vi "Handle Incoming Packets.vi"(8 "error in (no error)":errorcluster, 9 "SessionMailbox":refnum<queue>, 10 "Incoming Packet":refnum<class "ControlPacket.lvclass">, 11 "Server in":refnum<class "Server.lvclass">) -> (0 "error out":errorcluster, 1 "SessionMailbox out":refnum<queue>, 2 "Outgoing":T1, 3 "Server out":refnum<class "Server.lvclass">)   [LabVIEW 2013, in "MQTT Server.lvlib" / "Server.lvclass"]
uses:
  Server.lvclass
  Control Packets/ControlPacket/ControlPacket.lvclass
  MQTT_Base/Response -- cluster.ctl
  MQTT_Base/MQTT_Base.lvclass
  Control Packets/CONNECT/CONNECT.lvclass
  Control Packets/CONNACK/Connect Return Code -- enum.ctl
  Control Packets/PUBLISH/PUBLISH.lvclass
  Control Packets/ControlPacket/ControlPacket.lvclass/ControlPacket.ctl
  Control Packets/PUBREL/PUBREL.lvclass
  Control Packets/SUBSCRIBE/SUBSCRIBE.lvclass
  Control Packets/SUBACK/Subscription Success Code.ctl
  Control Packets/ControlPacket/QualityOfService -- enum.ctl
  Control Packets/UNSUBSCRIBE/UNSUBSCRIBE.lvclass
  Control Packets/PINGREQ/PINGREQ.lvclass
  Control Packets/CONNACK/CONNACK.lvclass
  Control Packets/PUBCOMP/PUBCOMP.lvclass
  Control Packets/SUBACK/SUBACK.lvclass
  Control Packets/PUBACK/PUBACK.lvclass
  Control Packets/PUBREC/PUBREC.lvclass
  Control Packets/PINGRESP/PINGRESP.lvclass
  Control Packets/UNSUBACK/UNSUBACK.lvclass
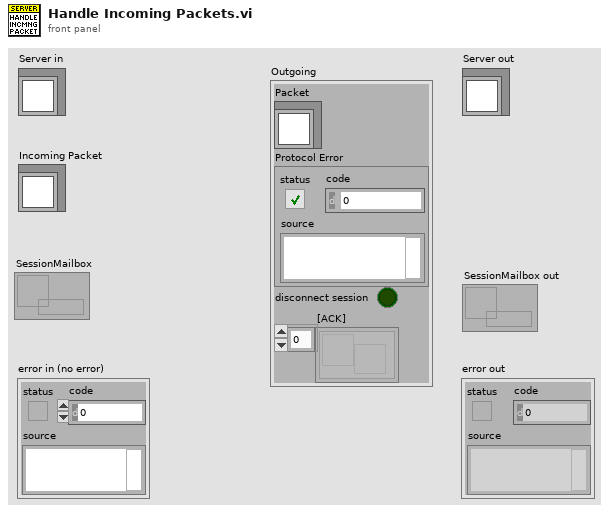
[diagram p1: front panel]
types:
  T1 = typedef "MQTT Server.lvlib/MQTT_Base.lvclass/Response -- cluster.ctl" = cluster{"Packet":refnum<class "ControlPacket.lvclass">, "Protocol Error":errorcluster, "disconnect session":bool, "[ACK]":refnum<notifier>[]}
  T2 = typedef "CONNACK.lvclass/Connect Return Code -- enum.ctl" = enum16{"Connection accepted", "Unacceptable protocol version", "Identifier Rejected", "Server Unavailable", "Bad Username or Password", "Not Authorized"}
  T3 = typedef "SUBACK.lvclass/Subscription Success Code.ctl" = cluster{"Subscription Failure":bool, "QoS":T4}
  T4 = typedef "ControlPacket.lvclass/QualityOfService -- enum.ctl" = enum16{"0 (At Most Once)", "1 (At Least Once)", "2 (Exactly Once)"}
  T5 = typedef "ControlPacket.lvclass/Control Packet Type -- enum.ctl" = enum16{"Reserved", "CONNECT", "CONNACK", "PUBLISH", "PUBACK", "PUBREC", "PUBREL", "PUBCOMP", "SUBSCRIBE", "SUBACK", "UNSUBSCRIBE", "UNSUBACK", "PINGREQ", "PINGRESP", "DISCONNECT", "Reserved(15)"}
  T6 = typedef "CONNECT.lvclass/ConnectFlags -- cluster.ctl" = cluster{"Reserved":bool, "Clean Session":bool, "Will Flag":bool, "Will QoS 1":bool, "Will QoS 2":bool, "Will Retain":bool, "Password Flag":bool, "User Name Flag":bool}
  T7 = typedef "CONNECT.lvclass/ConnectPayload -- cluster.ctl" = cluster{"Will Topic":string, "Will Message":string, "Username":string, "Password":string}
  T8 = typedef "SUBSCRIBE.lvclass/Topic Subscription -- cluster.ctl" = cluster{"Topic Filter":string, "QoS":T4}
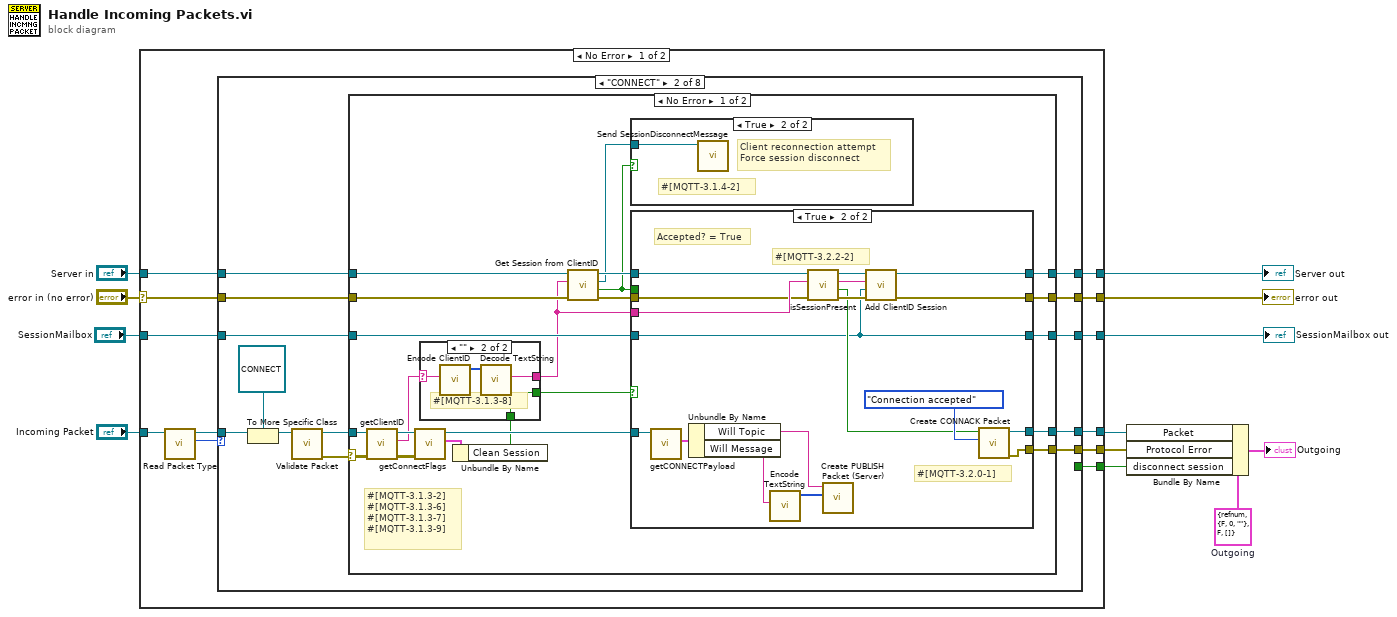
[diagram p0: block diagram]
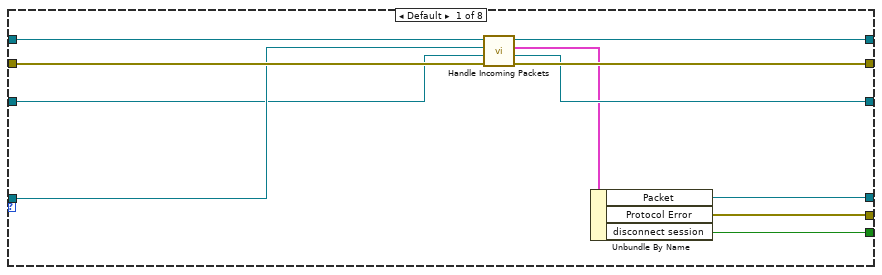
[diagram p2: hidden frame]
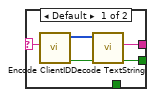
[diagram p3: hidden frame]
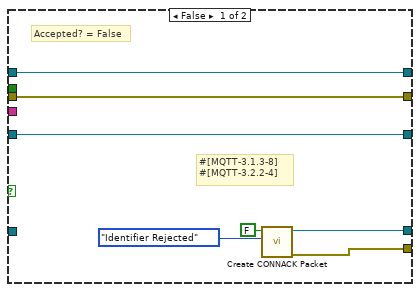
[diagram p5: hidden frame]
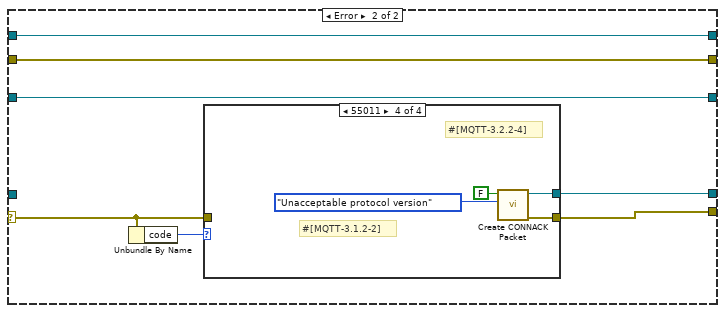
[diagram p6: hidden frame]
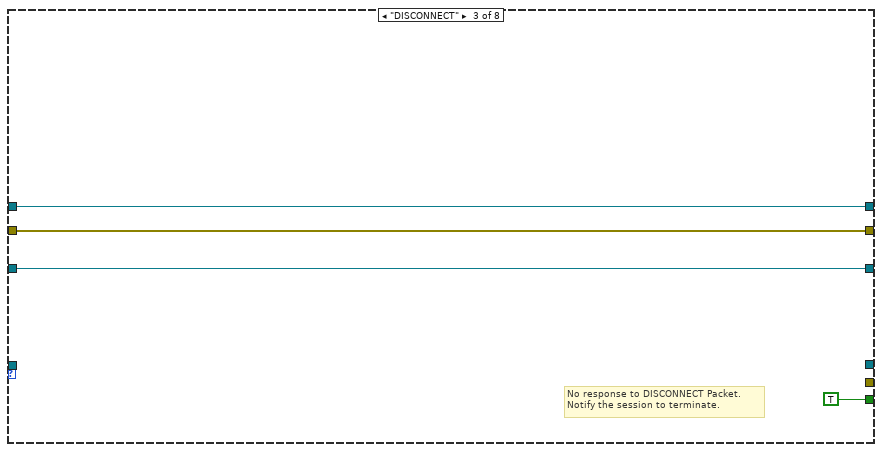
[diagram p10: hidden frame]
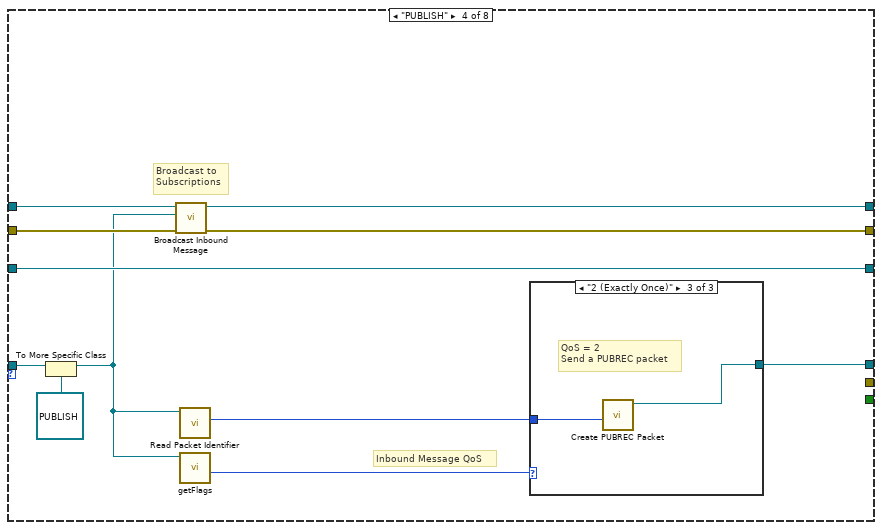
[diagram p11: hidden frame]
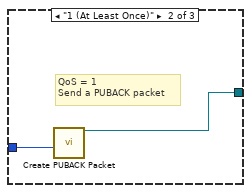
[diagram p13: hidden frame]
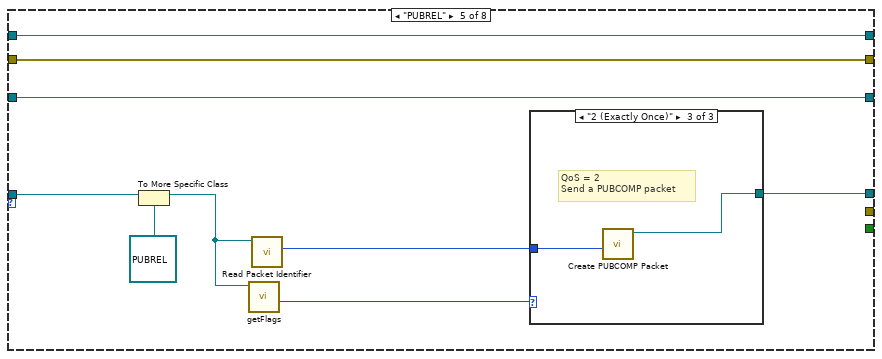
[diagram p14: hidden frame]
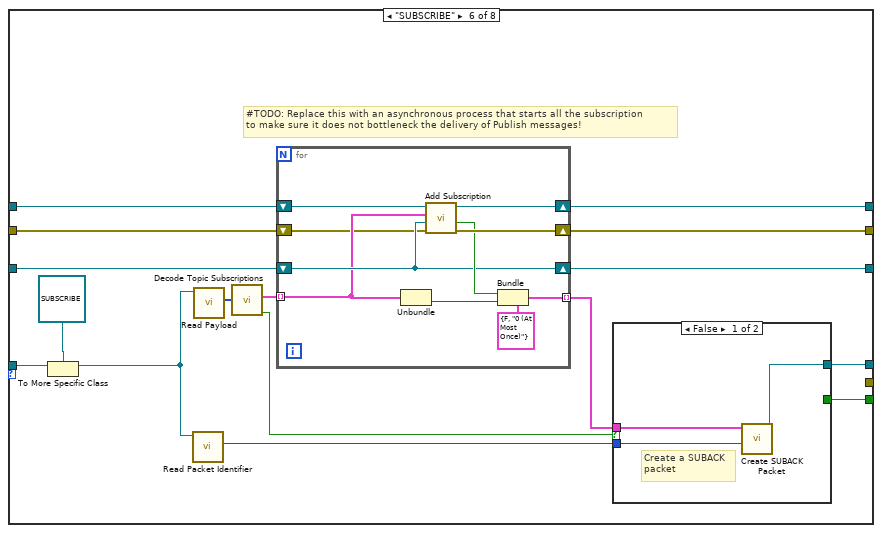
[diagram p17: hidden frame]
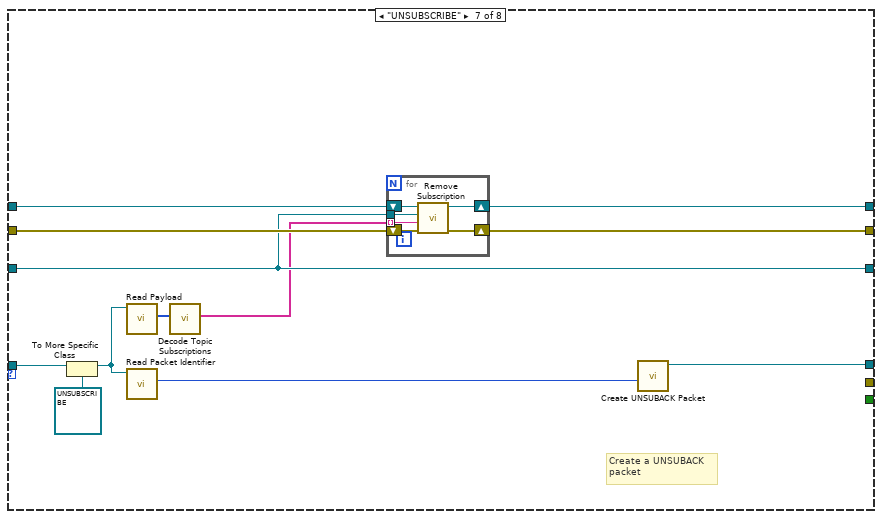
[diagram p19: hidden frame]
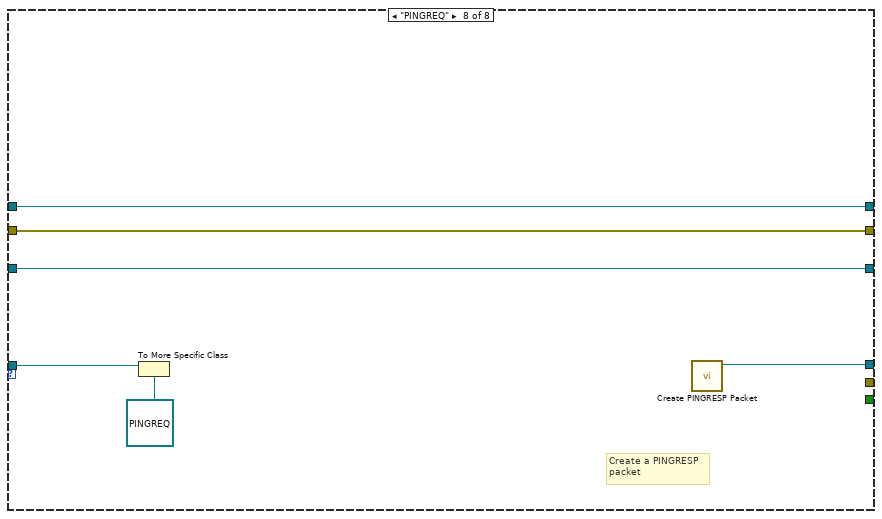
[diagram p20: hidden frame]
diagram:
  w7 = T1 {"Packet"=refnum, "Protocol Error"={"status"=FALSE, "code"=0, "source"=""}, "disconnect session"=FALSE, "[ACK]"=[]}  # Outgoing
  n1 = case shown="No Error" "error in (no error)" {
    selector: "error in (no error)" -> [w22 w203]
    tunnel: [w19 w203] -> w11
    tunnel: [w20 w202] -> w9
    tunnel: "Server in" -> [w21 w202]
    tunnel: "Incoming Packet" -> [w15 _]
    tunnel: [w18 _] -> w6
    tunnel: [w17 _] -> w2
    tunnel: "SessionMailbox" -> [w16 w201]
    tunnel: [w14 w201] -> w1
    tunnel: [w13 _] -> w4
    frame No Error {
      n2 = call "Read Packet Type.vi"("ControlPacket in"=w15) -> ("Control Packet Type"=w24:T5, "ControlPacket out"=w23:refnum<class "ControlPacket.lvclass">)  [unwired: 9 in]
      n3 = case shown="\"CONNECT\"" w24 {
        tunnel: w23 -> [w31 w45 _ w130 w141 w162 w188 w197]
        tunnel: w22 -> [w33 w42 w119 w125 w143 w152 w184 w199]
        tunnel: w21 -> [w35 w43 w120 w123 w144 w155 w182 w200]
        tunnel: [w34 w40 w120 w122 w144 w154 w181 w200] -> w20
        tunnel: [w32 w41 w119 w124 w143 w153 w183 w199] -> w19
        tunnel: w16 -> [w30 w39 w117 w131 w142 w151 w180 w198]
        tunnel: [w27 w38 _ w126 w139 w156 w178 w196] -> w18
        tunnel: [w26 w37 _ _ _ _ _ _] -> w17
        tunnel: [w29 w36 w117 w131 w142 w150 w180 w198] -> w14
        tunnel: [w25 _ TRUE ("disconnect") _ _ w148 _ _] -> w13
        frame Default {
          n4 = call-parent "Handle Incoming Packets.vi"("error in (no error)"=w33, "SessionMailbox"=w30, "Incoming Packet"=w31, "MQTT_Base in"=w35) -> ("error out"=w32:errorcluster, "SessionMailbox out"=w29:refnum<queue>, "Outgoing"=w28:T1, "MQTT_Base out"=w34:refnum<class "Server.lvclass">)  [unwired: 4 in]
          n5 = Unbundle By Name(w28) -> ("Packet"=w27:refnum<class "ControlPacket.lvclass">, "Protocol Error"=w26:errorcluster, "disconnect session"=w25:bool)
        }
        frame "CONNECT" {
          n6 = To More Specific Class(target class=refnum<class "CONNECT.lvclass"> refnum ("CONNECT.lvclass"), reference=w45) -> (specific class reference=w44:refnum<class "CONNECT.lvclass">)  [unwired: 1 in, 1 out]
          n7 = call "Validate Packet.vi"("ControlPacket in"=w44) -> ("error out"=w48:errorcluster, "ControlPacket out"=w47:refnum<class "CONNECT.lvclass">)  [unwired: 9 in]
          n8 = case shown="No Error" w48 {
            selector: w48 -> [_ w108]
            tunnel: w47 -> [w68 _]
            tunnel: w43 -> [w64 w107]
            tunnel: w42 -> [w62 w106]
            tunnel: [w66 w106] -> w41
            tunnel: [w67 w107] -> w40
            tunnel: w39 -> [w65 w103]
            tunnel: [w59 w105] -> w38
            tunnel: [w58 w104] -> w37
            tunnel: [w56 w103] -> w36
            frame No Error {
              # "#[MQTT-3.1.3-2]\n#[MQTT-3.1.3-6]\n#[MQTT-3.1.3-7]\n#[MQTT-3.1.3-9]"
              n9 = call "getClientID.vi"("CONNECT in"=w68) -> ("Client ID"=w50:string, "CONNECT out"=w55:refnum<class "CONNECT.lvclass">)  [unwired: 9 in]
              n10 = call "getConnectFlags.vi"("CONNECT in"=w55) -> ("Connect Flags"=w53:T6, "CONNECT out"=w54:refnum<class "CONNECT.lvclass">)  [unwired: 9 in]
              n11 = Unbundle By Name(w53) -> ("Clean Session"=w51:bool)
              n12 = case shown="\"\"" w50 {
                selector: w50 -> [w72 w75]
                tunnel: [w71 w76] -> w52
                tunnel: w51 -> [_ w76]
                tunnel: [w69 w73] -> w49
                frame Default {
                  n13 = call "Encode ClientID.vi"("Client ID (empty: generate new)"=w72) -> ("valid Client ID"=w71:bool, "Length-Prefixed Field"=w70:u8[])  [unwired: 9 in]
                  n14 = call "Decode TextString.vi"("Length-Prefixed Field"=w70) -> ("Text String"=w69:string)  [unwired: 8 in, 2 out]
                }
                frame "" {
                  # "#[MQTT-3.1.3-8]"
                  n15 = call "Encode ClientID.vi"("Client ID (empty: generate new)"=w75) -> ("Length-Prefixed Field"=w74:u8[])  [unwired: 9 in, 1 out]
                  n16 = call "Decode TextString.vi"("Length-Prefixed Field"=w74) -> ("Text String"=w73:string)  [unwired: 8 in, 2 out]
                }
              }
              n17 = call "Get Session from ClientID.vi"("error in (no error)"=w62, "Client ID"=w49, "MQTT_Base in"=w64) -> ("error out"=w61:errorcluster, "found?"=w57:bool, "SessionMailbox"=w60:refnum<queue>, "MQTT_Base out"=w63:refnum<class "Server.lvclass">)  [unwired: 5 in]
              n18 = case shown="True" w57 {
                tunnel: w60 -> [_ w77]
                frame False {
                }
                frame True {
                  # "#[MQTT-3.1.4-2]"
                  # "Client reconnection attempt\nForce session disconnect"
                  n19 = call "Send SessionDisconnectMessage.vi"("SessionMailbox"=w77) -> ()  [unwired: 10 in, 1 out]
                }
              }
              n20 = case shown="True" w52 {
                tunnel: [w82 w101] -> w67
                tunnel: [w81 w100] -> w66
                tunnel: w65 -> [w78 w90]
                tunnel: w63 -> [w82 w92]
                tunnel: w61 -> [w81 w91]
                tunnel: w49 -> [_ w96]
                tunnel: [w80 w99] -> w59
                tunnel: [w79 w98] -> w58
                tunnel: w57 -> [_ _]
                tunnel: [w78 w90] -> w56
                tunnel: w54 -> [_ w89]
                frame False {
                  # "Accepted? = False"
                  # "#[MQTT-3.1.3-8]\n#[MQTT-3.2.2-4]"
                  n21 = call "Create CONNACK Packet.vi"("Return Code"=Connect_Return_Code_--_enum."Identifier Rejected", "Session Present"=FALSE) -> ("error out"=w79:errorcluster, "CONNACK"=w80:refnum<class "CONNACK.lvclass">)  [unwired: 8 in]
                }
                frame True {
                  # "Accepted? = True"
                  # "#[MQTT-3.2.2-2]"
                  # "#[MQTT-3.2.0-1]"
                  n22 = call "getCONNECTPayload.vi"("CONNECT in"=w89) -> ("Payload"=w88:T7)  [unwired: 9 in, 1 out]
                  n23 = Unbundle By Name(w88) -> ("Will Topic"=w87:string, "Will Message"=w85:string)
                  n24 = call "Encode TextString.vi"("Text String"=w85) -> ("Length-Prefixed Field"=w86:u8[])  [unwired: 10 in]
                  n25 = call "isSessionPresent.vi"("error in"=w91, "Client ID"=w96, "MQTT_Base in"=w92) -> ("error out"=w97:errorcluster, "Session Present"=w94:bool, "Client ID dup"=w95:string, "MQTT_Base out"=w93:refnum<class "Server.lvclass">)  [unwired: 5 in]
                  n26 = call "Create PUBLISH Packet (Server).vi"("Payload"=w86, "Topic Name"=w87) -> ()  [unwired: 7 in, 3 out]
                  n27 = call "Add ClientID Session.vi"("error in (no error)"=w97, "SessionMailbox"=w90, "Client ID"=w95, "MQTT_Base in"=w93) -> ("error out"=w100:errorcluster, "MQTT_Base out"=w101:refnum<class "Server.lvclass">)  [unwired: 6 in]
                  n28 = call "Create CONNACK Packet.vi"("Return Code"=Connect_Return_Code_--_enum."Connection accepted", "Session Present"=w94) -> ("error out"=w98:errorcluster, "CONNACK"=w99:refnum<class "CONNACK.lvclass">)  [unwired: 8 in]
                }
              }
            }
            frame Error {
              n29 = Unbundle By Name(w108) -> ("code"=w109:i32)
              n30 = case shown="55011" w109 {
                tunnel: [_ _ _ w114] -> w105
                tunnel: [w110 w111 w112 w113] -> w104
                tunnel: w108 -> [w110 w111 w112 _]
                frame Default {
                  # "#[MQTT-3.1.4-1]"
                  # "Any unhandled error should be\nthralled to the Protocol error terminal"
                }
                frame 55010 {
                  # "#[MQTT-3.1.2-1]"
                }
                frame 55012 {
                  # "#[MQTT-3.1.2-3]"
                }
                frame 55011 {
                  # "#[MQTT-3.2.2-4]"
                  # "#[MQTT-3.1.2-2]"
                  n31 = call "Create CONNACK Packet.vi"("Return Code"=Connect_Return_Code_--_enum."Unacceptable protocol version", "Session Present"=FALSE) -> ("error out"=w113:errorcluster, "CONNACK"=w114:refnum<class "CONNACK.lvclass">)  [unwired: 8 in]
                }
              }
            }
          }
        }
        frame "DISCONNECT" {
          # "No response to DISCONNECT Packet.\nNotify the session to terminate."
        }
        frame "PUBLISH" {
          # "Broadcast to\nSubscriptions"
          # "Inbound Message QoS"
          n32 = To More Specific Class(target class=refnum<class "PUBLISH.lvclass"> refnum ("PUBLISH.lvclass"), reference=w130) -> (specific class reference=w121:refnum<class "PUBLISH.lvclass">)  [unwired: 1 in, 1 out]
          n33 = call "Broadcast Inbound Message.vi"("error in (no error)"=w125, "Inbound Message"=w121, "MQTT_Base in"=w123) -> ("error out"=w124:errorcluster, "MQTT_Base out"=w122:refnum<class "Server.lvclass">)  [unwired: 7 in]
          n34 = call "Read Packet Identifier.vi"("ControlPacket in"=w121) -> ("Packet Identifier"=w127:u16)  [unwired: 9 in, 1 out]
          n35 = call-dynamic "getFlags.vi"("PUBLISH in"=w121) -> ("QoS"=w128:T4)  [unwired: 7 in, 3 out]
          n36 = case shown="\"2 (Exactly Once)\"" w128 {
            tunnel: w127 -> [_ w133 w135]
            tunnel: [_ w132 w134] -> w126
            frame "0 (At Most Once)", Default {
            }
            frame "1 (At Least Once)" {
              # "QoS = 1\nSend a PUBACK packet"
              n37 = call "Create PUBACK Packet.vi"("Packet ID"=w133) -> ("PUBACK out"=w132:refnum<class "PUBACK.lvclass">)  [unwired: 9 in, 1 out]
            }
            frame "2 (Exactly Once)" {
              # "QoS = 2\nSend a PUBREC packet"
              n38 = call "Create PUBREC Packet.vi"("Packet ID"=w135) -> ("PUBREC out"=w134:refnum<class "PUBREC.lvclass">)  [unwired: 9 in, 1 out]
            }
          }
        }
        frame "PUBREL" {
          n39 = To More Specific Class(target class=refnum<class "PUBREL.lvclass"> refnum ("PUBREL.lvclass"), reference=w141) -> (specific class reference=w137:refnum<class "PUBREL.lvclass">)  [unwired: 1 in, 1 out]
          n40 = call-dynamic "getFlags.vi"("PUBREL in"=w137) -> ("QoS"=w136:T4)  [unwired: 7 in, 3 out]
          n41 = call "Read Packet Identifier.vi"("ControlPacket in"=w137) -> ("Packet Identifier"=w140:u16)  [unwired: 9 in, 1 out]
          n42 = case shown="\"2 (Exactly Once)\"" w136 {
            tunnel: w140 -> [_ _ w146]
            tunnel: [_ _ w145] -> w139
            frame "0 (At Most Once)", Default {
            }
            frame "1 (At Least Once)" {
            }
            frame "2 (Exactly Once)" {
              # "QoS = 2\nSend a PUBCOMP packet"
              n43 = call "Create PUBCOMP Packet.vi"("Packet ID"=w146) -> ("PUBCOMP out"=w145:refnum<class "PUBCOMP.lvclass">)  [unwired: 9 in, 1 out]
            }
          }
        }
        frame "SUBSCRIBE" {
          # "#TODO: Replace this with an asynchronous process that starts all the subscription\nto make sure it does not bottleneck the delivery of Publish messages!"
          n44 = To More Specific Class(target class=refnum<class "SUBSCRIBE.lvclass"> refnum ("SUBSCRIBE.lvclass"), reference=w162) -> (specific class reference=w147:refnum<class "SUBSCRIBE.lvclass">)  [unwired: 1 in, 1 out]
          n45 = call "Read Packet Identifier.vi"("ControlPacket in"=w147) -> ("Packet Identifier"=w159:u16)  [unwired: 9 in, 1 out]
          n46 = call "Read Payload.vi"("ControlPacket in"=w147) -> ("Payload"=w160:u8[])  [unwired: 9 in, 1 out]
          n47 = call "Decode Topic Subscriptions.vi"("Payload"=w160) -> ("invalid UTF8"=w149:bool, "Topic Subscriptions"=w158:T8[])  [unwired: 8 in, 1 out]
          n48 = for {
            tunnel: w158 -> [w169] mode=indexing
            tunnel: [w176] -> w157 mode=indexing
            shift-right: [w172] -> w154
            shift-left: w155 -> [w168]
            shift-right: [w173] -> w153
            shift-left: w152 -> [w167]
            shift-right: [w170] -> w150
            shift-left: w151 -> [w170]
            n49 = Unbundle(w169) -> ("QoS"=w174:T4)  [unwired: 1 out]
            n50 = call "Add Subscription.vi"("error in (no error)"=w167, "SessionMailbox"=w170, "Topic Subscription"=w169, "MQTT_Base in"=w168) -> ("error out"=w173:errorcluster, "Failed"=w171:bool, "MQTT_Base out"=w172:refnum<class "Server.lvclass">)  [unwired: 5 in]
            n51 = Bundle(cluster=T3 {"Subscription Failure"=FALSE, "QoS"=enum."0 (At Most Once)"} ("Topic Subscription"), "Subscription Failure"=w171, "QoS"=w174) -> (w176:T3)
          }
          n52 = case shown="False" w149 {
            selector: w149 -> [_ w166]
            tunnel: w159 -> [w165 _]
            tunnel: w157 -> [w164 _]
            tunnel: [w163 _] -> w156
            tunnel: [_ w166] -> w148
            frame False {
              # "Create a SUBACK\npacket"
              n53 = call "Create SUBACK Packet.vi"("Packet ID"=w165, "Return Codes"=w164) -> ("SUBACK"=w163:refnum<class "SUBACK.lvclass">)  [unwired: 8 in, 1 out]
            }
            frame True {
              # "Invalid UTF8 string"
            }
          }
        }
        frame "UNSUBSCRIBE" {
          # "Create a UNSUBACK\npacket"
          n54 = To More Specific Class(target class=refnum<class "UNSUBSCRIBE.lvclass"> refnum ("UNSUBSCRIBE.lvclass"), reference=w188) -> (specific class reference=w187:refnum<class "UNSUBSCRIBE.lvclass">)  [unwired: 1 in, 1 out]
          n55 = call "Read Payload.vi"("ControlPacket in"=w187) -> ("Payload"=w185:u8[])  [unwired: 9 in, 1 out]
          n56 = call "Read Packet Identifier.vi"("ControlPacket in"=w187) -> ("Packet Identifier"=w177:u16)  [unwired: 9 in, 1 out]
          n57 = call "Decode Topic Subscriptions.vi"("Payload"=w185) -> ("Topic Subscriptions"=w179:string[])  [unwired: 9 in, 1 out]
          n58 = for {
            tunnel: w180 -> [w190]
            shift-right: [w191] -> w181
            shift-left: w182 -> [w192]
            shift-right: [w193] -> w183
            shift-left: w184 -> [w194]
            tunnel: w179 -> [w189] mode=indexing
            n59 = call "Remove Subscription.vi"("error in (no error)"=w194, "Topic Filter"=w189, "SessionMailbox"=w190, "MQTT_Base in"=w192) -> ("error out"=w193:errorcluster, "MQTT_Base out"=w191:refnum<class "Server.lvclass">)  [unwired: 5 in, 1 out]
          }
          n60 = call "Create UNSUBACK Packet.vi"("Packet ID"=w177) -> ("UNSUBACK out"=w178:refnum<class "UNSUBACK.lvclass">)  [unwired: 9 in, 1 out]
        }
        frame "PINGREQ" {
          # "Create a PINGRESP\npacket"
          n61 = To More Specific Class(target class=refnum<class "PINGREQ.lvclass"> refnum ("PINGREC.lvclass"), reference=w197) -> ()  [unwired: 1 in, 2 out]
          n62 = call "Create PINGRESP Packet.vi"() -> ("PINGRESP out"=w196:refnum<class "PINGRESP.lvclass">)  [unwired: 10 in, 1 out]
        }
      }
    }
    frame Error {
    }
  }
  "error out" <- w11
  "Server out" <- w9
  "SessionMailbox out" <- w1
  n63 = Bundle By Name(cluster=w7, "Packet"=w6, "Protocol Error"=w2, "disconnect session"=w4) -> (→"Outgoing":T1)
